vi "Static Channel Lookup.vi"(8 "error in (no error)":errorcluster, 11 "Device Item Ref in":T1 format="%.0x") -> (0 "error out":errorcluster, 2 "Configuration Data":T2, 3 "Item Ref out":T1=18446744073709551615 format="%.0x")   [LabVIEW 2015, in "SLSC Module Template System Explorer.lvlib"]
uses:
  SLSC Module Template System Explorer.lvlib
  <vilib>/NI Veristand/Custom Device API/Custom Device Item Ref.ctl
  Shared/Compiled.Settings
  Shared/SLSC Dynamic Channel.ctl
  Shared/Constants.vi
  <vilib>/NI Veristand/Custom Device API/Get Item Property (Variant).vi
  <vilib>/regexp/Match Regular Expression.xnode
  Shared/SLSC Module Template Shared.lvlib
  <vilib>/NI Veristand/Custom Device API/Custom Device API.lvlib
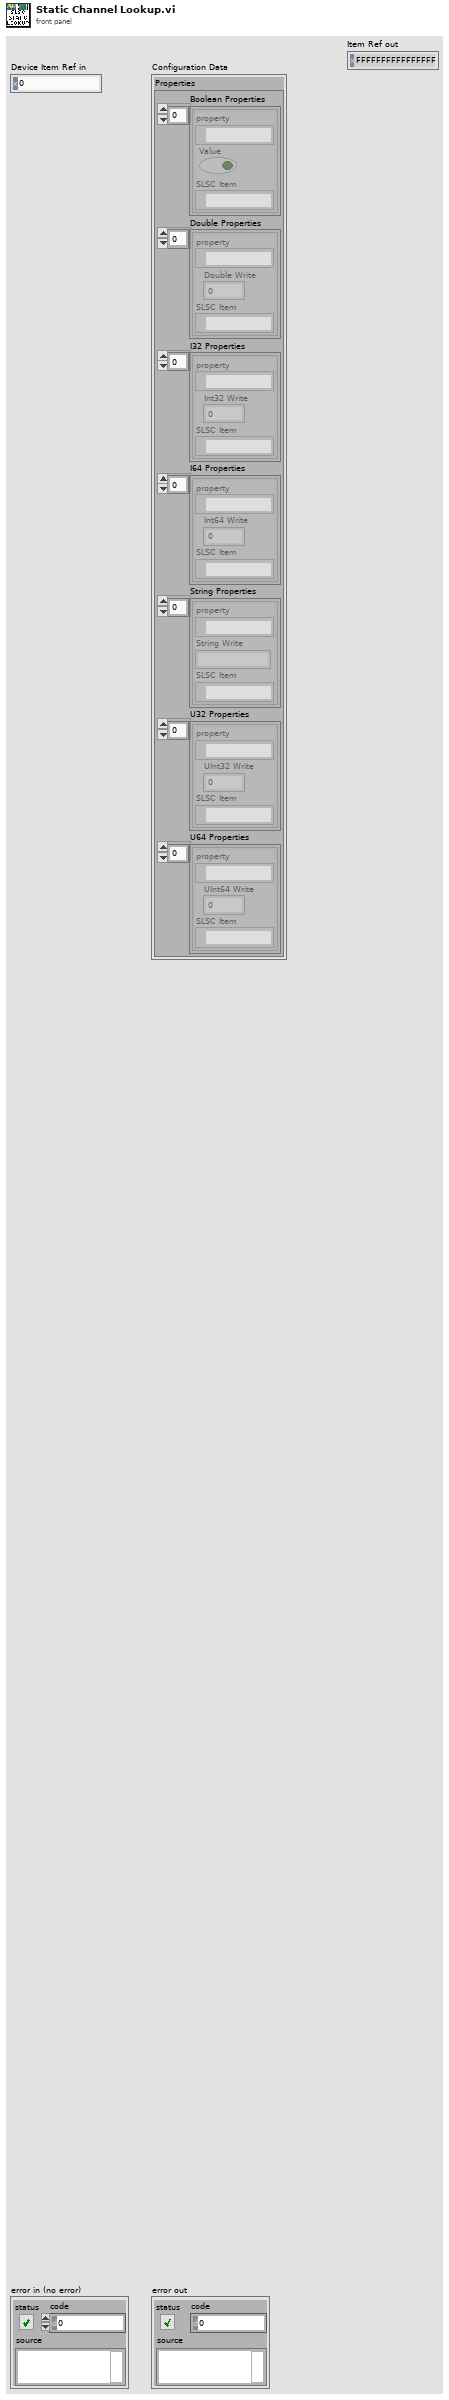
[diagram p1: front panel]
types:
  T1 = typedef "Custom Device API.lvlib/Custom Device Item Ref.ctl" = u64
  T2 = cluster{"Properties":cluster{"Boolean Properties":cluster{"property":refnum<k21>, "Value":bool, "SLSC Item":refnum<k21>}[], "Double Properties":cluster{"property":refnum<k21>, "Double Write":dbl, "SLSC Item":refnum<k21>}[], "I32 Properties":cluster{"property":refnum<k21>, "Int32 Write":i32, "SLSC Item":refnum<k21>}[], "I64 Properties":cluster{"property":refnum<k21>, "Int64 Write":i64, "SLSC Item":refnum<k21>}[], "String Properties":cluster{"property":refnum<k21>, "String Write":string, "SLSC Item":refnum<k21>}[], "U32 Properties":cluster{"property":refnum<k21>, "UInt32 Write":u32, "SLSC Item":refnum<k21>}[], "U64 Properties":cluster{"property":refnum<k21>, "UInt64 Write":u64, "SLSC Item":refnum<k21>}[]}}
  T3 = typedef "SLSC Module Template Shared.lvlib/Compiled.Settings" = cluster{"Name":string, "SLSC IP Address":string, "Slot #":i32, "Configuration Data":cluster{"Properties":cluster{"Boolean Properties":cluster{"property":refnum<k21>, "Value":bool, "SLSC Item":refnum<k21>}[], "Double Properties":cluster{"property":refnum<k21>, "Double Write":dbl, "SLSC Item":refnum<k21>}[], "I32 Properties":cluster{"property":refnum<k21>, "Int32 Write":i32, "SLSC Item":refnum<k21>}[], "I64 Properties":cluster{"property":refnum<k21>, "Int64 Write":i64, "SLSC Item":refnum<k21>}[], "String Properties":cluster{"property":refnum<k21>, "String Write":string, "SLSC Item":refnum<k21>}[], "U32 Properties":cluster{"property":refnum<k21>, "UInt32 Write":u32, "SLSC Item":refnum<k21>}[], "U64 Properties":cluster{"property":refnum<k21>, "UInt64 Write":u64, "SLSC Item":refnum<k21>}[]}}, "SLSC Dynamic Inputs":T4[], "SLSC Dynamic Outputs":T4[], "SLSC Dynamic Commands":T4[]}
  T4 = typedef "SLSC Module Template System Explorer.lvlib/SLSC Dynamic Channel.ctl" = cluster{"SLSC Item":string, "property":string, "Data Type":enum16{"Bool", "Double", "I32", "I64", "String", "U32", "U64"}}
  T5 = cluster{"property":refnum<k21>, "Value":bool, "SLSC Item":refnum<k21>}
  T6 = cluster{"property":refnum<k21>, "Double Write":dbl, "SLSC Item":refnum<k21>}
  T7 = cluster{"property":refnum<k21>, "Int32 Write":i32, "SLSC Item":refnum<k21>}
  T8 = cluster{"property":refnum<k21>, "Int64 Write":i64, "SLSC Item":refnum<k21>}
  T9 = cluster{"property":refnum<k21>, "String Write":string, "SLSC Item":refnum<k21>}
  T10 = cluster{"property":refnum<k21>, "UInt32 Write":u32, "SLSC Item":refnum<k21>}
  T11 = cluster{"property":refnum<k21>, "UInt64 Write":u64, "SLSC Item":refnum<k21>}
  T12 = cluster{"property":refnum<k21>, "Value":bool, "SLSC Item":refnum<k21>}[]
  T13 = cluster{"property":refnum<k21>, "Double Write":dbl, "SLSC Item":refnum<k21>}[]
  T14 = cluster{"property":refnum<k21>, "Int32 Write":i32, "SLSC Item":refnum<k21>}[]
  T15 = cluster{"property":refnum<k21>, "Int64 Write":i64, "SLSC Item":refnum<k21>}[]
  T16 = cluster{"property":refnum<k21>, "String Write":string, "SLSC Item":refnum<k21>}[]
  T17 = cluster{"property":refnum<k21>, "UInt32 Write":u32, "SLSC Item":refnum<k21>}[]
  T18 = cluster{"property":refnum<k21>, "UInt64 Write":u64, "SLSC Item":refnum<k21>}[]
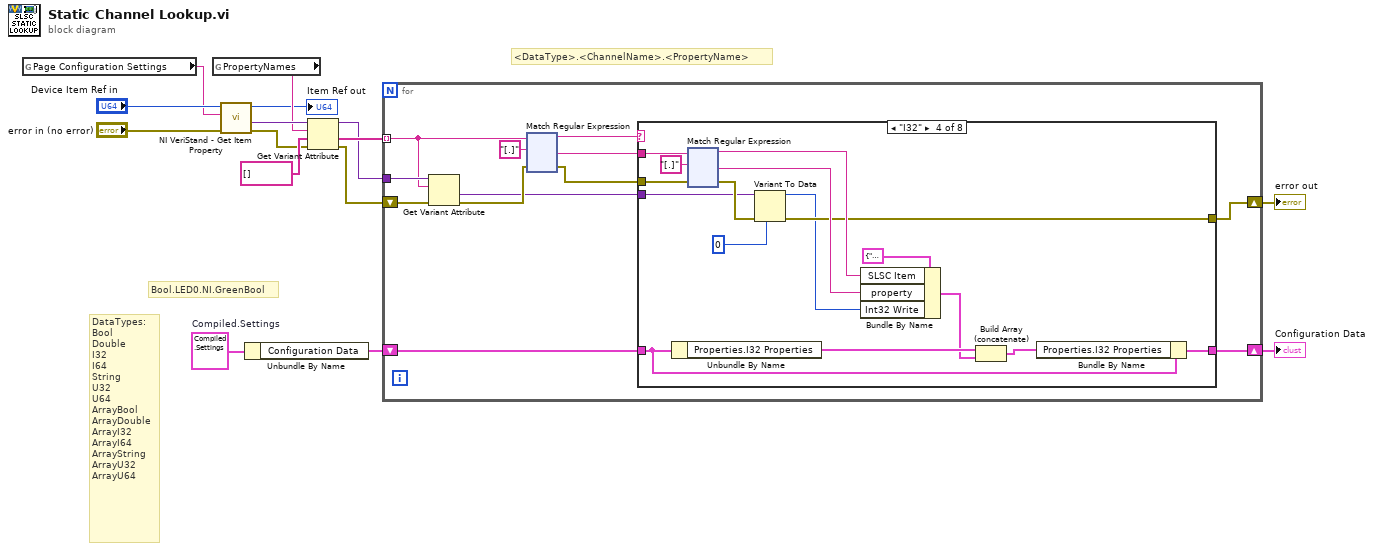
[diagram p0: block diagram]
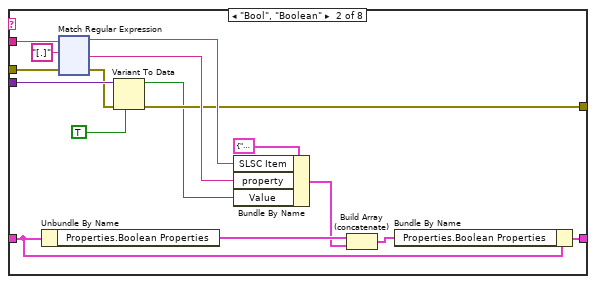
[diagram p3: hidden frame]
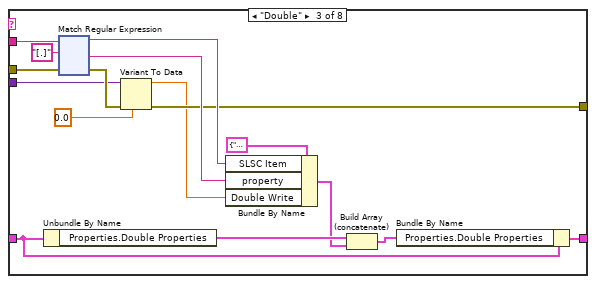
[diagram p4: hidden frame]
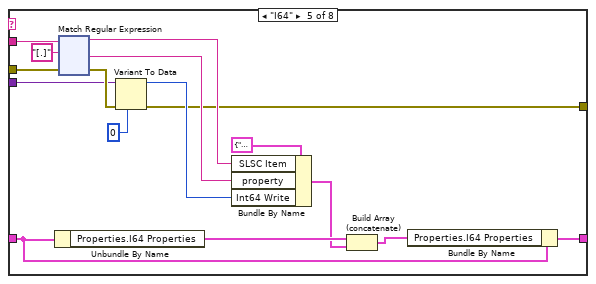
[diagram p5: hidden frame]
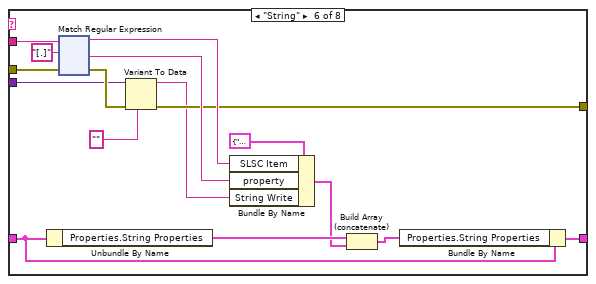
[diagram p6: hidden frame]
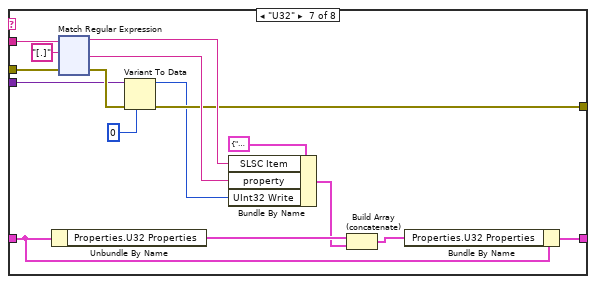
[diagram p7: hidden frame]
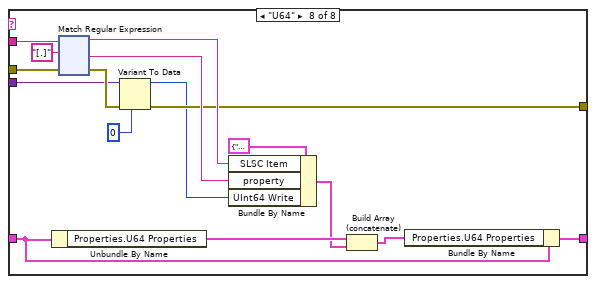
[diagram p8: hidden frame]
diagram:
  w13 = T3 {"Name"="", "SLSC IP Address"="", "Slot #"=0, "Configuration Data"={"Properties"={"Boolean Properties"=[], "Double Properties"=[], "I32 Properties"=[], "I64 Properties"=[], "String Properties"=[], "U32 Properties"=[], "U64 Properties"=[]}}, "SLSC Dynamic Inputs"=[], "SLSC Dynamic Outputs"=[], "SLSC Dynamic Commands"=[]}  # Compiled.Settings
  # "DataTypes:\nBool\nDouble\nI32\nI64\nString\nU32\nU64\nArrayBool\nArrayDouble\nArrayI32\nArrayI64\nArrayString\nArrayU32\nArrayU64"
  # "Bool.LED0.NI.GreenBool"
  # "<DataType>.<ChannelName>.<PropertyName>"
  n1 = global read "Constants.vi" "Page Configuration Settings"() -> (w3:string)
  n2 = global read "Constants.vi" "PropertyNames"() -> (w2:string)
  n3 = call-poly <vilib>:"NI VeriStand - Get Item Property.vi"("error in (no error)"="error in (no error)", "Property Name"=w3, "Item Ref in"="Device Item Ref in") -> ("error out"=w5:errorcluster, "Value"=w9:variant, "Item Ref out"=→"Item Ref out":T1)  [unwired: 5 in, 1 out]
  n4 = Unbundle By Name(w13) -> ("Configuration Data"=w10:T2)
  n5 = Get Variant Attribute(Variant=w9, name=w2, default value (empty Variant)=string[] [], error in=w5) -> (duplicate Variant=w6:variant, value=w7:string[], error out=w4:errorcluster)  [unwired: 1 out]
  n6 = for {
    shift-right: [w25] -> w14
    shift-left: w4 -> [w18]
    shift-right: [w27] -> w15
    shift-left: w10 -> [w26]
    tunnel: w7 -> [w19] mode=indexing
    tunnel: w6 -> [w20]
    n7 = Get Variant Attribute(Variant=w20, name=w19, error in=w18) -> (value=w16:variant, error out=w17:errorcluster)  [unwired: 1 in, 2 out]
    n8 = xnode "Match Regular Expression"("input string"=w19, "regular expression"="[.]", "error in"=w17) -> ("before match"=w23:string, "after match"=w22:string, "error out"=w21:errorcluster)  [unwired: 3 in, 2 out]
    n9 = case shown="\"I32\"" w23 {
      tunnel: w22 -> [_ w44 w174 w304 w434 w564 w694 w824]
      tunnel: w21 -> [w28 w43 w173 w303 w433 w563 w693 w823]
      tunnel: w26 -> [w29 w30 w168 w290 w420 w550 w680 w810]
      tunnel: [w29 w36 w166 w297 w427 w557 w687 w817] -> w27
      tunnel: [w28 w32 w163 w293 w424 w553 w684 w814] -> w25
      tunnel: w16 -> [_ w34 w161 w291 w422 w551 w682 w811]
      frame Default {
      }
      frame "Bool", "Boolean" {
        n10 = Unbundle By Name(w30) -> ("Properties.Boolean Properties"=w39:T12)
        n11 = xnode "Match Regular Expression"("input string"=w44, "regular expression"="[.]", "error in"=w43) -> ("before match"=w41:string, "after match"=w40:string, "error out"=w33:errorcluster)  [unwired: 3 in, 2 out]
        n12 = Variant To Data(error in=w33, type=TRUE, Variant=w34) -> (data=w31:bool, error out=w32:errorcluster)
        n13 = Bundle By Name(cluster=T5 {"property"="", "Value"=FALSE, "SLSC Item"=""} ("Device and Property"), "SLSC Item"=w41, "property"=w40, "Value"=w31) -> (w38:T5)
        n14 = Build Array (concatenate)(w39, w38) -> (w37:T12)
        n15 = Bundle By Name(cluster=w30, "Properties.Boolean Properties"=w37) -> (w36:T2)
      }
      frame "Double" {
        n16 = Unbundle By Name(w168) -> ("Properties.Double Properties"=w170:T13)
        n17 = xnode "Match Regular Expression"("input string"=w174, "regular expression"="[.]", "error in"=w173) -> ("before match"=w172:string, "after match"=w171:string, "error out"=w164:errorcluster)  [unwired: 3 in, 2 out]
        n18 = Variant To Data(error in=w164, type=0.0, Variant=w161) -> (data=w162:dbl, error out=w163:errorcluster)
        n19 = Bundle By Name(cluster=T6 {"property"="", "Double Write"=0.0, "SLSC Item"=""} ("Device and Property"), "SLSC Item"=w172, "property"=w171, "Double Write"=w162) -> (w169:T6)
        n20 = Build Array (concatenate)(w170, w169) -> (w167:T13)
        n21 = Bundle By Name(cluster=w168, "Properties.Double Properties"=w167) -> (w166:T2)
      }
      frame "I32" {
        n22 = Unbundle By Name(w290) -> ("Properties.I32 Properties"=w300:T14)
        n23 = xnode "Match Regular Expression"("input string"=w304, "regular expression"="[.]", "error in"=w303) -> ("before match"=w302:string, "after match"=w301:string, "error out"=w294:errorcluster)  [unwired: 3 in, 2 out]
        n24 = Variant To Data(error in=w294, type=0, Variant=w291) -> (data=w292:i32, error out=w293:errorcluster)
        n25 = Bundle By Name(cluster=T7 {"property"="", "Int32 Write"=0, "SLSC Item"=""} ("Device and Property 2"), "SLSC Item"=w302, "property"=w301, "Int32 Write"=w292) -> (w299:T7)
        n26 = Build Array (concatenate)(w300, w299) -> (w298:T14)
        n27 = Bundle By Name(cluster=w290, "Properties.I32 Properties"=w298) -> (w297:T2)
      }
      frame "I64" {
        n28 = Unbundle By Name(w420) -> ("Properties.I64 Properties"=w430:T15)
        n29 = xnode "Match Regular Expression"("input string"=w434, "regular expression"="[.]", "error in"=w433) -> ("before match"=w432:string, "after match"=w431:string, "error out"=w423:errorcluster)  [unwired: 3 in, 2 out]
        n30 = Variant To Data(error in=w423, type=i64 0, Variant=w422) -> (data=w425:i64, error out=w424:errorcluster)
        n31 = Bundle By Name(cluster=T8 {"property"="", "Int64 Write"=0, "SLSC Item"=""} ("Device and Property 2"), "SLSC Item"=w432, "property"=w431, "Int64 Write"=w425) -> (w429:T8)
        n32 = Build Array (concatenate)(w430, w429) -> (w428:T15)
        n33 = Bundle By Name(cluster=w420, "Properties.I64 Properties"=w428) -> (w427:T2)
      }
      frame "String" {
        n34 = Unbundle By Name(w550) -> ("Properties.String Properties"=w560:T16)
        n35 = xnode "Match Regular Expression"("input string"=w564, "regular expression"="[.]", "error in"=w563) -> ("before match"=w562:string, "after match"=w561:string, "error out"=w555:errorcluster)  [unwired: 3 in, 2 out]
        n36 = Variant To Data(error in=w555, type="", Variant=w551) -> (data=w552:string, error out=w553:errorcluster)
        n37 = Bundle By Name(cluster=T9 {"property"="", "String Write"="", "SLSC Item"=""} ("Device and Property 2"), "SLSC Item"=w562, "property"=w561, "String Write"=w552) -> (w559:T9)
        n38 = Build Array (concatenate)(w560, w559) -> (w558:T16)
        n39 = Bundle By Name(cluster=w550, "Properties.String Properties"=w558) -> (w557:T2)
      }
      frame "U32" {
        n40 = Unbundle By Name(w680) -> ("Properties.U32 Properties"=w690:T17)
        n41 = xnode "Match Regular Expression"("input string"=w694, "regular expression"="[.]", "error in"=w693) -> ("before match"=w692:string, "after match"=w691:string, "error out"=w685:errorcluster)  [unwired: 3 in, 2 out]
        n42 = Variant To Data(error in=w685, type=u32 0, Variant=w682) -> (data=w683:u32, error out=w684:errorcluster)
        n43 = Bundle By Name(cluster=T10 {"property"="", "UInt32 Write"=0, "SLSC Item"=""} ("Device and Property 2"), "SLSC Item"=w692, "property"=w691, "UInt32 Write"=w683) -> (w689:T10)
        n44 = Build Array (concatenate)(w690, w689) -> (w688:T17)
        n45 = Bundle By Name(cluster=w680, "Properties.U32 Properties"=w688) -> (w687:T2)
      }
      frame "U64" {
        n46 = Unbundle By Name(w810) -> ("Properties.U64 Properties"=w820:T18)
        n47 = xnode "Match Regular Expression"("input string"=w824, "regular expression"="[.]", "error in"=w823) -> ("before match"=w822:string, "after match"=w821:string, "error out"=w815:errorcluster)  [unwired: 3 in, 2 out]
        n48 = Variant To Data(error in=w815, type=u64 0, Variant=w811) -> (data=w812:u64, error out=w814:errorcluster)
        n49 = Bundle By Name(cluster=T11 {"property"="", "UInt64 Write"=0, "SLSC Item"=""} ("Device and Property 2"), "SLSC Item"=w822, "property"=w821, "UInt64 Write"=w812) -> (w819:T11)
        n50 = Build Array (concatenate)(w820, w819) -> (w818:T18)
        n51 = Bundle By Name(cluster=w810, "Properties.U64 Properties"=w818) -> (w817:T2)
      }
    }
  }
  "Configuration Data" <- w15
  "error out" <- w14
